vi "memory_load_MLP_1_B_1.vi"() -> (0 "Init Data Out":fxp<+/-,32,16>)   [LabVIEW 2020]
panel:
  # "For Initialization VI requirements and help, please read directions located on Block Diagram."
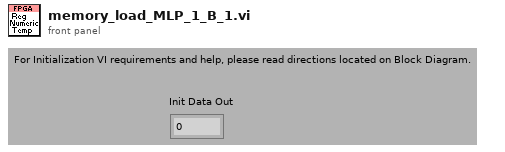
[diagram p1: front panel]
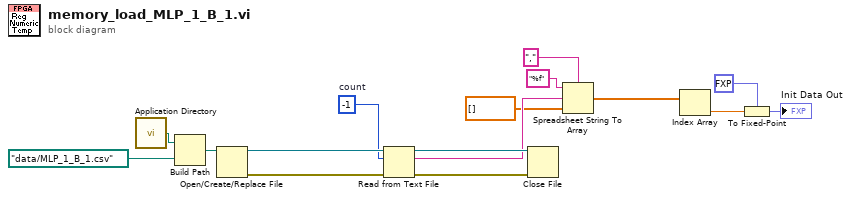
[diagram p0: block diagram]
diagram:
  w4 = -1  # count
  n1 = call <vilib>:"Application Directory.vi"() -> ("Application Directory"=w8:path)
  n2 = Build Path(base path=w8, name or relative path=path "data/MLP_1_B_1.csv" ("default name")) -> (appended path=w7:path)
  n3 = Open/Create/Replace File(file path (use dialog)=w7) -> (refnum out=w12:refnum<file>, error out=w13:errorcluster)  [unwired: 5 in, 1 out]
  n4 = Read from Text File(file (use dialog)=w12, count=w4, error in=w13) -> (refnum out=w11:refnum<file>, text=w9:string, error out=w10:errorcluster)  [unwired: 1 in, 1 out]
  n5 = Close File(refnum=w11, error in=w10) -> ()  [unwired: 2 out]
  n6 = Spreadsheet String To Array(delimiter (Tab)=",", format string="%f", spreadsheet string=w9, array type (2D Dbl)=dbl[] []) -> (array=w1:dbl[])
  n7 = Index Array(array=w1) -> (element=w15:dbl)  [unwired: 1 in]
  n8 = To Fixed-Point(fixed-point type=fxp<+/-,32,16> 0.0 ("fixed-point"), number=w15) -> (fixed-point=→"Init Data Out":fxp<+/-,32,16>)
